vi "PopUp_Select Shared Resource.vi"(8 "error in (no error)":errorcluster, 11 "*ResData":refnum<data-value>) -> (0 "error out":errorcluster, 2 "OK Pressed?":bool, 3 "Resource":T1)   [LabVIEW 2013, in "SET Project Editor.lvlib"]
uses:
  SET Project Editor.lvlib
  SET Project Data/Resource Data Class/Resource Data.lvclass
  SET Project Data/Types/ProjFile_Resource Entry.ctl
  DialogEnum.ctl
  SET Project Data/Resource Data Class/Resource Data.lvclass/Resource Data.ctl
  SET Project Data/Resource Data Class/Read Shared Resources.vi
  SET Project Data/Resource Data Class/Read Languages.vi
  SET Project Data/SET Project Data.lvlib
panel:
  in  "Resources":i32(listbox)
  in  "Cancel":bool
  in  "OK":bool
  # "Select Resource"
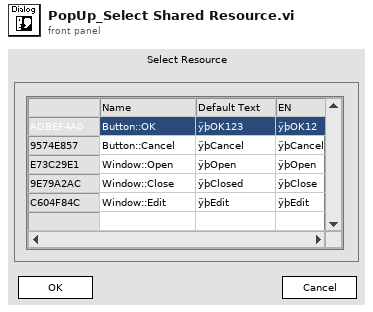
[diagram p1: front panel]
types:
  T1 = typedef "SET Project Data.lvlib/ProjFile_Resource Entry.ctl" = cluster{"RID":string, "Tag":string, "Strings [] (UTF-16)":string[], "Shared?":bool}
  T2 = typedef "SET Project Editor.lvlib/DialogEnum.ctl" = enum16{"Idle", "Init", "Shutdown"}
  T3 = typedef "SET Project Data.lvlib/ProjFile_Resource Data.ctl" = cluster{"RID":string, "Tag":string, "Strings [] (UTF-16)":string[], "Shared?":bool}
  T4 = typedef "SET Project Data.lvlib/ProjFile_Language Data.ctl" = cluster{"Tag":string, "Name":string, "Code Page":u16}
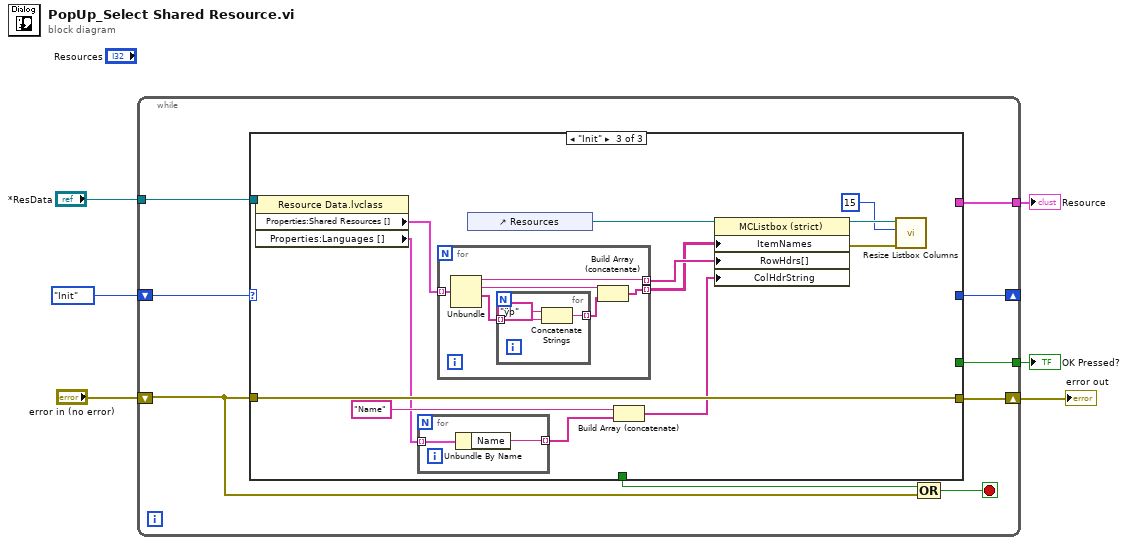
[diagram p0: block diagram]
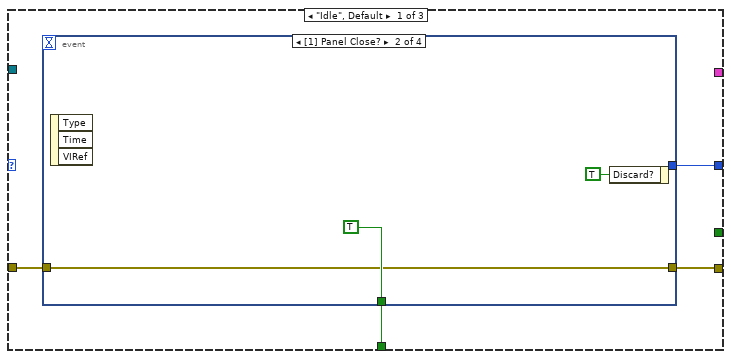
[diagram p2: hidden frame]
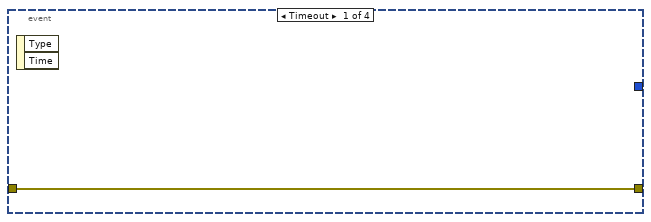
[diagram p3: hidden frame]
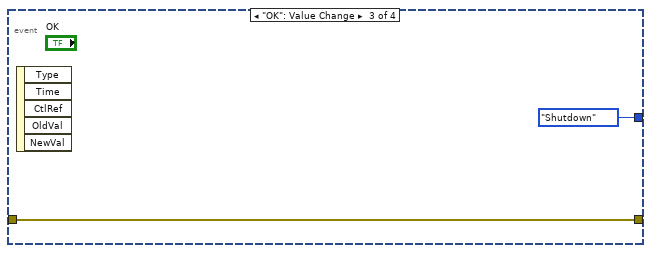
[diagram p4: hidden frame]
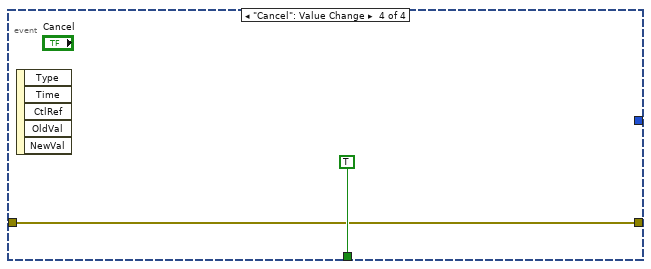
[diagram p5: hidden frame]
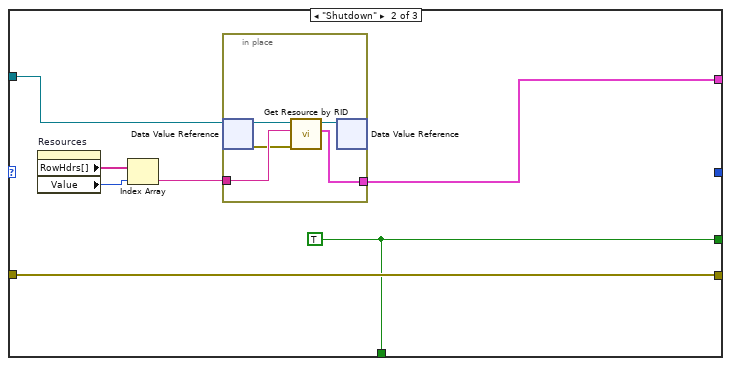
[diagram p6: hidden frame]
diagram:
  n1 = while {
    shift-right: [w14] -> w4
    shift-left: "error in (no error)" -> [w11]
    shift-right: [w13] -> _
    shift-left: DialogEnum."Init" -> [w15]
    tunnel: "*ResData" -> [w9]
    tunnel: [w8] -> w2
    tunnel: [w7] -> w1
    stop <- w10 stop-if-true
    n2 = case shown="\"Init\"" w15 {
      tunnel: [w19 w34 w52] -> w14
      tunnel: w11 -> [w18 w34 w52]
      tunnel: [w17 w28 _] -> w12
      tunnel: [w16 _ _] -> w13
      tunnel: w9 -> [_ w33 w51]
      tunnel: [_ w29 _] -> w8
      tunnel: [_ w28 _] -> w7
      frame "Idle", Default {
        n3 = event shown="[1] Panel Close?" {
          selector: _ -> [_ _ _ _]
          dyn-events: _ -> [_ _ _ _]
          timeout: _ -> [_ _ _ _]
          tunnel: [w20 w21 w24 w26] -> w19
          tunnel: w18 -> [w20 w21 w24 w26]
          tunnel: [_ TRUE _ TRUE] -> w17
          tunnel: [_ _ DialogEnum."Shutdown" _] -> w16
          event Timeout {
            n4 = event-data() -> ()  [unwired: 1 in, 2 out]
          }
          event Panel Close? {
            n5 = event-data() -> ()  [unwired: 1 in, 3 out]
            n6 = event-data("Discard?"=TRUE) -> ()  [unwired: 1 in, 1 out]
          }
          event "OK": Value Change {
            n7 = event-data() -> ()  [unwired: 1 in, 5 out]
          }
          event "Cancel": Value Change {
            n8 = event-data() -> ()  [unwired: 1 in, 5 out]
          }
        }
      }
      frame "Shutdown" {
        w28 = TRUE
        n9 = property on="Resources" class="MCListbox (strict)"() -> ("RowHdrs[]"=w32:string[], "Value"=w31:i32)  [unwired: 2 in, 2 out]
        n10 = Index Array(array=w32, index=w31) -> (element=w30:string)
        n11 = in-place {
          in-place-border: w30 -> [w38]
          in-place-border: [w35] -> w29
          n12 = in-place-dvr #1(w33) -> (w39:refnum<class "Resource Data.lvclass">, w37:errorcluster)
          n13 = call "Get Resource by RID.vi"("error in (no error)"=w37, "RID"=w38, "LangFile in"=w39) -> ("Resource"=w35:T1, "LangFile out"=w36:refnum<class "Resource Data.lvclass">)  [unwired: 4 in, 3 out]
          n14 = in-place-dvr #1(w36) -> ()  [unwired: 2 out]
        }
      }
      frame "Init" {
        n15 = property class="Resource Data.lvclass"(reference=w51) -> ("Properties:Shared Resources []"=w50:T3[], "Properties:Languages []"=w41:T4[])  [unwired: 1 in, 2 out]
        n16 = for {
          tunnel: w41 -> [w54] mode=indexing
          tunnel: [w53] -> w40 mode=indexing
          n17 = Unbundle By Name(w54) -> ("Name"=w53:string)
        }
        n18 = for {
          tunnel: w50 -> [w60] mode=indexing
          tunnel: [w59] -> w44 mode=indexing
          tunnel: [w57] -> w42 mode=indexing
          n19 = Unbundle(w60) -> ("RID"=w59:string, "Tag"=w58:string, "Strings [] (UTF-16)"=w56:string[])  [unwired: 1 out]
          n20 = for {
            tunnel: w56 -> [w63] mode=indexing
            tunnel: [w62] -> w55 mode=indexing
            n21 = Concatenate Strings("ÿþ" ("string"), w63) -> (w62:string)
          }
          n22 = Build Array (concatenate)(w58, w55) -> (w57:string[])
        }
        n23 = control-ref of="Resources"() -> (w45:refnum<vi>)
        n24 = Build Array (concatenate)("Name", w40) -> (w43:string[])
        n25 = property class="MCListbox (strict)"(reference=w45, "ItemNames"=w42, "RowHdrs[]"=w44, "ColHdrString"=w43) -> (reference out=w47:refnum<vi>, error out=w48:errorcluster)  [unwired: 1 in]
        n26 = call "Resize Listbox Columns.vi"("error in (no error)"=w48, "Padding (5px)"=i16 15, "Listbox Control ref in"=w47) -> ()  [unwired: 7 in, 2 out]
      }
    }
    n27 = Compound Arithmetic op=OR(w12, w11) -> (w10:bool)
  }
  "error out" <- w4
  "Resource" <- w2
  "OK Pressed?" <- w1
